vi "emi_Bool Changed w init.vi"(7 "x":bool, 13 "Initial(F)":bool) -> (6 "Rising":bool, 8 "changed":bool, 10 "Falling":bool)   [LabVIEW 2011]
doc: "Monitors a bool, indicateing change, and wheter it was rising or falling. \n\nFirst call will always give out false on all outputs, asuming the previous is the same as the first.\n\nreentrant Subroutine."
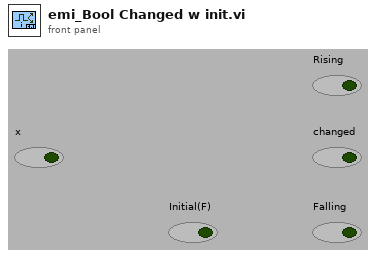
[diagram p1: front panel]
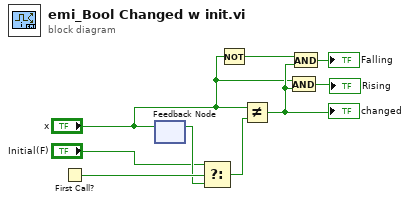
[diagram p0: block diagram]
diagram:
  n1 = First Call?() -> (First Call?: T/F=w9:bool)
  n2 = feedback-in #1("x") -> ()
  n3 = feedback #1() -> (w8:bool)  [unwired: 1 in]
  n4 = Select(t="Initial(F)", s=w9, f=w8) -> (s? t:f=w7:bool)
  n5 = Not(x="x") -> (.not. x?=w4:bool)
  n6 = Not Equal?(x="x", y=w7) -> (x != y?=w3:bool)
  "changed" <- w3
  n7 = And(x="x", y=w3) -> (x .and. y?=→"Rising":bool)
  n8 = And(x=w4, y=w3) -> (x .and. y?=→"Falling":bool)
